vi "setDACLimits.vi"(8 "error in":T3, 10 "DAC":T1 items=["DAC 1", "DAC 2", "DAC 3", "DAC 4"], 11 "DAC-Limits":T2={"Current Limit"=-inf, "LT-Limit"=-inf, "RT-Limit"=-inf} {"RT-Limit" format="%#_g V"; "LT-Limit" format="%#_g V"; "Current Limit" format="%#_g V"}) -> (0 "error out":T3, 3 "DAC-Limits out":T2={"Current Limit"=-inf, "LT-Limit"=-inf, "RT-Limit"=-inf} {"RT-Limit" format="%#_g V"; "LT-Limit" format="%#_g V"; "Current Limit" format="%#_g V"})   [LabVIEW 2016]
doc: "Sets the DAC limits. These values restrict the values that can be set with the setDAC.vi."
uses:
  Controls/Error_Out.ctl
  Controls/DAC_Limits.ctl
  Controls/DAC_Selection.ctl
  Files_ASC500/DLL/ASC500_RemoteControlV27.dll
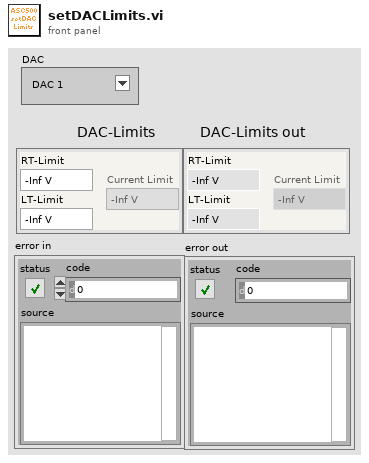
[diagram p1: front panel]
types:
  T1 = typedef "DAC_Selection.ctl" = u16
  T2 = typedef "DAC_Limits.ctl" = cluster{"Current Limit":sgl, "LT-Limit":sgl, "RT-Limit":sgl}
  T3 = typedef "Error_Out.ctl" = errorcluster
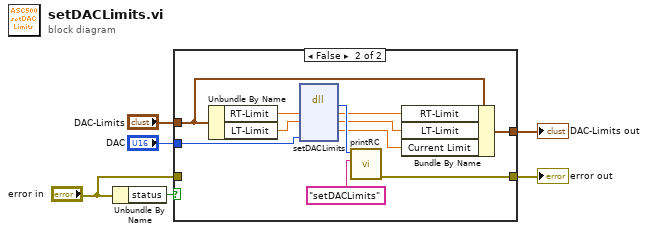
[diagram p0: block diagram]
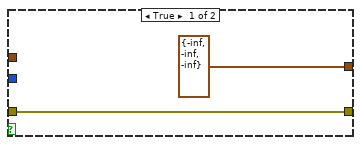
[diagram p2: hidden frame]
diagram:
  n1 = Unbundle By Name("error in") -> ("status"=w4:bool)
  n2 = case shown="False" w4 {
    tunnel: [w8 w18] -> w5
    tunnel: "error in" -> [w8 _]
    tunnel: "DAC-Limits" -> [_ w11]
    tunnel: [T2 {"Current Limit"=-inf, "LT-Limit"=-inf, "RT-Limit"=-inf} ("DAC-Limits out 2") w10] -> w2
    tunnel: "DAC" -> [_ w9]
    frame True {
    }
    frame False {
      n3 = Unbundle By Name(w11) -> ("RT-Limit"=w16:sgl, "LT-Limit"=w15:sgl)
      n4 = dll-call lib="G:/SCMOperations/Share/ELE/Produkt Information/ASC500/04 Remote Control/02 development versions/2018Nov06/Files_ASC500/DLL/ASC500_RemoteControlV27.dll" fn="setDACLimits"("RTLimit"=w16, "LTLimit"=w15, "DAC"=w9) -> ("return type"=w19:i32, "RTLimit"=w14:sgl, "LTLimit"=w13:sgl, "CurrentDACLimit"=w12:sgl)  [unwired: 5 in, 2 out]
      n5 = call "printRC.vi"("additional information"="setDACLimits", "RC"=w19) -> ("error out"=w18:T3)  [unwired: 9 in]
      n6 = Bundle By Name(cluster=w11, "RT-Limit"=w14, "LT-Limit"=w13, "Current Limit"=w12) -> (w10:T2)
    }
  }
  "error out" <- w5
  "DAC-Limits out" <- w2
